vi "Get Frequency Shift.vi"(0 "niUsrpRio session":T1 {"Daughterboard Clock Rate" format="%#.3pHz"; "FPGA Data Clock Rate" format="%#.3pHz"; "Data Clock Rate" format="%#.3pHz"; "Characterization Data"."Frequencies [Hz]" format="%#_6p"; "EEPROM Characterization Header"."Pointer to Device Data Header" format="%x"; "EEPROM Characterization Header"."Checksum" format="%x"; "Device Data Header"."Pointer to Characterization Data" format="%x"; "Device Data Header"."Checksum" format="%x"; "EEPROM Header"."Pointer to User Header" format="%x"; "EEPROM Header"."Pointer to Factory Header" format="%x"; "EEPROM Header"."Product Code" format="%x"; "EEPROM Header"."Checksum" format="%x"}, 1 "scope":string(combo)="rx/RF 0", 11 "error in":errorcluster) -> (4 "niUsrpRio Session (out)":T1={"FPGA Interface"=refnum, "RIO Interface Number"=0, "Data Clock Rate"=0, "FPGA Data Clock Rate"=0, "Global Settings Register Bus"=refnum, "Radio 0 Settings Register Bus"=refnum, "Radio 1 Settings Register Bus"=refnum, "Radio Settings Bus Semaphore"=refnum, "DB Queues"=[], "Characterization Data Valid?"=FALSE, "EEPROM Header"={"Checksum"=0, "Product Code"=0, "Hardware Current Version"=0, "Hardware Oldest Compatible Version"=0, "EEPROM Map Current Version"=0, "EEPROM Map Oldest Compatible Version"=0, "User Password"="", "Pointer to Factory Header"=0, "Pointer to User Header"=0, "Recommended Interval"=0, "Number of Reserved Bytes"=9, "Number of Daughterboards"=0, "Daughterboard IDs"=[], "Daughterboard Serial Numbers"=[]}, "Device Data Header"={"Checksum"=0, "Number of Channels"=0, "Number of Gain Settings"=[], "Pointer to Characterization Data"=[], "Number of Reserved Bytes"=27, "Number of Frequencies"=[]}, "EEPROM Characterization Header"={"Checksum"=0, "Date"=timestamp(0 s since 1904-01-01), "Temperature"=0.0, "Misc. Info"="", "Pointer to Device Data Header"=0, "Number of Reserved Bytes"=28}, "Characterization Data"=[], "FPGA Current Version"=0, "FPGA Oldest Compatible Version"=0, "Fixed Logic Current Version"=0, "Fixed Logic Oldest Compatible Version"=0, "FPGA Radio Settings Bus Current Version"=0, "FPGA Radio Settings Bus Oldest Compatible Version"=0, "FPGA Board Config Current Version"=0, "FPGA Board Config Oldest Compatible Version"=0, "Daughterboard Clock Rate"=0, "daughterboard configuration session handles"=[]} {"Daughterboard Clock Rate" format="%#.3pHz"; "FPGA Data Clock Rate" format="%#.3pHz"; "Data Clock Rate" format="%#.3pHz"; "Characterization Data"."Frequencies [Hz]" format="%#_6p"; "EEPROM Characterization Header"."Pointer to Device Data Header" format="%x"; "EEPROM Characterization Header"."Checksum" format="%x"; "Device Data Header"."Pointer to Characterization Data" format="%x"; "Device Data Header"."Checksum" format="%x"; "EEPROM Header"."Pointer to User Header" format="%x"; "EEPROM Header"."Pointer to Factory Header" format="%x"; "EEPROM Header"."Product Code" format="%x"; "EEPROM Header"."Checksum" format="%x"}, 6 "frequency shift":dbl format="%#.3pHz", 15 "error out":errorcluster)   [LabVIEW 2018]
uses:
  <instrlib>/niUsrpRio/Config/v1/Host/Public/niUsrpRio Session.ctl
  <instrlib>/_niInstr/Register Bus/v0/Host/Public/Register Bus Session.ctl
  <instrlib>/_niInstr/Register Bus/v0/Host/Private/Session Data.ctl
  <instrlib>/niUsrpRio/Config/v1/Host/Private/DB Queue Reference.ctl
  <instrlib>/niUsrpRio/Config/v1/Host/Private/Daughterboard Data.ctl
  <instrlib>/niUsrpRio/Config/v1/Host/Private/ATR state data.ctl
  <instrlib>/niUsrpRio/Config/v1/Host/Private/Antenna Configuration.ctl
  <instrlib>/niUsrpRio/Config/v1/Host/Private/CPLD Power Mode.ctl
  <instrlib>/niUsrpRio/Config/v1/Host/Public/EEPROM Header.ctl
  <instrlib>/niUsrpRio/Config/v1/Host/Public/EEPROM Device Data Header.ctl
  <instrlib>/niUsrpRio/Config/v1/Host/Public/EEPROM Characterization Header.ctl
  <instrlib>/niUsrpRio/Config/v1/Host/Public/Characterization Data.ctl
  <instrlib>/niUsrpRio/Config/v1/Host/Public/IQ Imbalance.ctl
  Streaming Xvcr FPGA Ref.ctl
  <vilib>/Utility/error.llb/Error Cluster From Error Code.vi
  <vilib>/rvi/errors/niLvFpgaAdjustHostInterfaceError.vi
  <vilib>/ErrorRing/Error Ring.xnode
  <vilib>/rvi/interface/nirviReadWriteControl/nirviReadWriteControl.xnode
  <vilib>/rvi/interface/Simulation/niFpgaSimulationCallBeginRW.vi
  NiFpgaLv.dll
  <instrlib>/niUsrpRio/Config/v1/Host/niUsrpRio Config v1 Host.lvlib
  <instrlib>/_niInstr/Register Bus/v0/Host/niInstr Register Bus v0 Host.lvlib
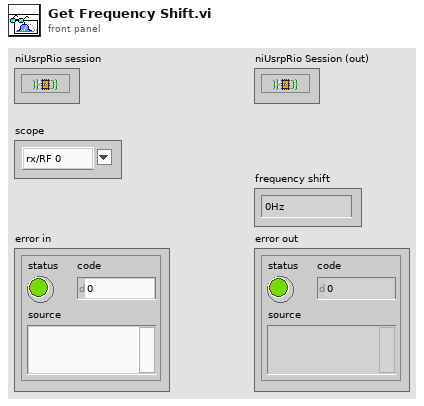
[diagram p1: front panel]
types:
  T1 = typedef "niUsrpRio Config v1 Host.lvlib/niUsrpRio Session.ctl" = cluster{"FPGA Interface":refnum<k20>, "RIO Interface Number":u32, "Data Clock Rate":u32, "FPGA Data Clock Rate":u32, "Global Settings Register Bus":T2, "Radio 0 Settings Register Bus":T2, "Radio 1 Settings Register Bus":T2, "Radio Settings Bus Semaphore":T3, "DB Queues":T4[], "Characterization Data Valid?":bool, "EEPROM Header":T5, "Device Data Header":T6, "EEPROM Characterization Header":T7, "Characterization Data":T8[], "FPGA Current Version":u32, "FPGA Oldest Compatible Version":u32, "Fixed Logic Current Version":u32, "Fixed Logic Oldest Compatible Version":u32, "FPGA Radio Settings Bus Current Version":u32, "FPGA Radio Settings Bus Oldest Compatible Version":u32, "FPGA Board Config Current Version":u32, "FPGA Board Config Oldest Compatible Version":u32, "Daughterboard Clock Rate":u32, "daughterboard configuration session handles":u64[]}
  T2 = typedef "niInstr Register Bus v0 Host.lvlib/Register Bus Session.ctl" = refnum<queue>
  T3 = typedef "Semaphore RefNum" = refnum<k1>
  T4 = typedef "niUsrpRio Config v1 Host.lvlib/DB Queue Reference.ctl" = refnum<queue>
  T5 = typedef "niUsrpRio Config v1 Host.lvlib/EEPROM Header.ctl" = cluster{"Checksum":u32, "Product Code":u16, "Hardware Current Version":u16, "Hardware Oldest Compatible Version":u16, "EEPROM Map Current Version":u16, "EEPROM Map Oldest Compatible Version":u16, "User Password":string, "Pointer to Factory Header":u32, "Pointer to User Header":u32, "Recommended Interval":u16, "Number of Reserved Bytes":i32, "Number of Daughterboards":u8, "Daughterboard IDs":u16[], "Daughterboard Serial Numbers":string[]}
  T6 = typedef "niUsrpRio Config v1 Host.lvlib/EEPROM Device Data Header.ctl" = cluster{"Checksum":u32, "Number of Channels":u8, "Number of Gain Settings":u16[], "Pointer to Characterization Data":u32[], "Number of Reserved Bytes":i32, "Number of Frequencies":u16[]}
  T7 = typedef "niUsrpRio Config v1 Host.lvlib/EEPROM Characterization Header.ctl" = cluster{"Checksum":u32, "Date":timestamp, "Temperature":sgl, "Misc. Info":string, "Pointer to Device Data Header":u32, "Number of Reserved Bytes":i32}
  T8 = typedef "niUsrpRio Config v1 Host.lvlib/Characterization Data.ctl" = cluster{"Gains[dB]":dbl[], "Frequencies [Hz]":dbl[], "IQ Imbalance Table":T9[], "Measured Gains[dB]":dbl[][]}
  T9 = typedef "niUsrpRio Config v1 Host.lvlib/IQ Imbalance.ctl" = cluster{"Gain Imbalance [linear]":dbl, "Phase Imbalance [radians]":dbl, "Offset":cdb}
  T10 = typedef "Streaming Xvcr FPGA Ref.ctl" = refnum<k20>
  T11 = typedef "niUsrpRio Config v1 Host.lvlib/Device Subfunction.ctl" = enum16{"rx", "tx", "all"}
  T12 = typedef "niUsrpRio Config v1 Host.lvlib/RF Channel 2.ctl" = enum16{"0", "1", "2", "3", "All"}
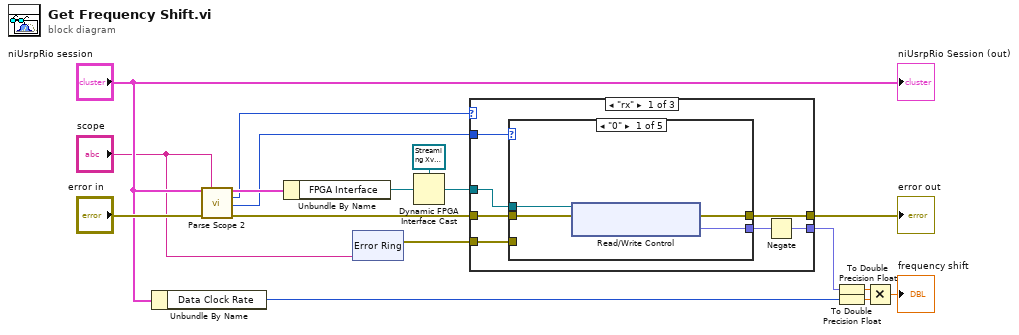
[diagram p0: block diagram]
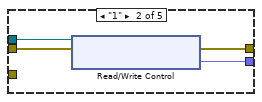
[diagram p2: hidden frame]
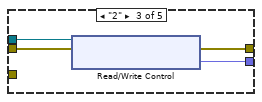
[diagram p3: hidden frame]
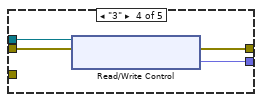
[diagram p4: hidden frame]
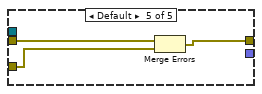
[diagram p5: hidden frame]
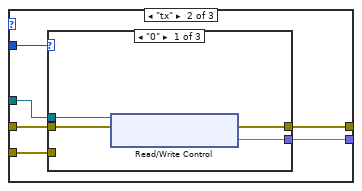
[diagram p6: hidden frame]
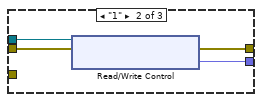
[diagram p7: hidden frame]
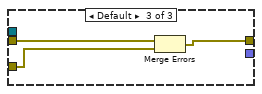
[diagram p8: hidden frame]
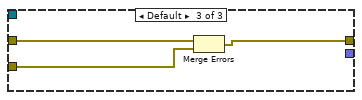
[diagram p9: hidden frame]
diagram:
  n1 = Unbundle By Name("niUsrpRio session") -> ("Data Clock Rate"=w3:u32)
  n2 = call <instrlib>:"Parse Scope 2.vi"("niUsrpRio Session"="niUsrpRio session", "scope"="scope", "error in"="error in") -> ("niUsrpRio Session (out)"=w17:T1, "Device Subfunction"=w9:T11, "Device Subfunction Channel"=w16:T12, "error out"=w10:errorcluster)  [unwired: 4 in, 5 out]
  n3 = Unbundle By Name(w17) -> ("FPGA Interface"=w13:refnum<k20>)
  n4 = xnode "Error Ring"("parameter 0"="scope") -> ("error out"=w2:errorcluster)
  n5 = Dynamic FPGA Interface Cast(Session In=T10 refnum ("FPGA VI Reference Out"), Type=w13) -> (Session Out=w12:T10)
  n6 = case shown="\"rx\"" w9 {
    tunnel: w12 -> [w21 w49 _]
    tunnel: [w24 w48 w62] -> w15
    tunnel: w10 -> [w23 w47 w63]
    tunnel: w16 -> [w22 w46 _]
    tunnel: [w19 w45 _] -> w6
    tunnel: w2 -> [w18 w44 w61]
    frame "rx" {
      n7 = case shown="\"0\"" w22 {
        tunnel: w21 -> [w28 w32 w36 w40 _]
        tunnel: [w27 w31 w35 w39 w42] -> w24
        tunnel: w23 -> [w26 w30 w34 w38 w43]
        tunnel: [w25 w29 w33 w37 _] -> w20
        tunnel: w18 -> [_ _ _ _ w41]
        frame "0" {
          n8 = xnode "Read/Write Control"("FPGA VI Reference In"=w28, "error in"=w26) -> ("error out"=w27:errorcluster, "rx 0.frequency shift"=w25:fxp<+/-,48,0>)  [unwired: 1 out]
        }
        frame "1" {
          n9 = xnode "Read/Write Control"("FPGA VI Reference In"=w32, "error in"=w30) -> ("error out"=w31:errorcluster, "rx 1.frequency shift"=w29:fxp<+/-,48,0>)  [unwired: 1 out]
        }
        frame "2" {
          n10 = xnode "Read/Write Control"("FPGA VI Reference In"=w36, "error in"=w34) -> ("error out"=w35:errorcluster, "rx 2.frequency shift"=w33:fxp<+/-,48,0>)  [unwired: 1 out]
        }
        frame "3" {
          n11 = xnode "Read/Write Control"("FPGA VI Reference In"=w40, "error in"=w38) -> ("error out"=w39:errorcluster, "rx 3.frequency shift"=w37:fxp<+/-,48,0>)  [unwired: 1 out]
        }
        frame Default {
          n12 = Merge Errors(w43, w41) -> (w42:errorcluster)
        }
      }
      n13 = Negate(x=w20) -> (-x=w19:fxp<+/-,49,1>)
    }
    frame "tx" {
      n14 = case shown="\"0\"" w46 {
        tunnel: w49 -> [w53 w57 _]
        tunnel: [w52 w56 w60] -> w48
        tunnel: w47 -> [w51 w55 w59]
        tunnel: [w50 w54 _] -> w45
        tunnel: w44 -> [_ _ w58]
        frame "0" {
          n15 = xnode "Read/Write Control"("FPGA VI Reference In"=w53, "error in"=w51) -> ("error out"=w52:errorcluster, "tx 0.frequency shift"=w50:fxp<+/-,48,0>)  [unwired: 1 out]
        }
        frame "1" {
          n16 = xnode "Read/Write Control"("FPGA VI Reference In"=w57, "error in"=w55) -> ("error out"=w56:errorcluster, "tx 1.frequency shift"=w54:fxp<+/-,48,0>)  [unwired: 1 out]
        }
        frame Default {
          n17 = Merge Errors(w59, w58) -> (w60:errorcluster)
        }
      }
    }
    frame Default {
      n18 = Merge Errors(w63, w61) -> (w62:errorcluster)
    }
  }
  "error out" <- w15
  n19 = To Double Precision Float(number=w6) -> (double precision float=w7:dbl)
  n20 = To Double Precision Float(number=w3) -> (double precision float=w4:dbl)
  n21 = Multiply(x=w7, y=w4) -> (x*y=→"frequency shift":dbl)
  "niUsrpRio Session (out)" <- "niUsrpRio session"
